vi "Read & Graph Measurement File.vi"() -> ()   [LabVIEW 2019]
panel:
  in  "File 2":path=path "test.tdms" caption="Filename"
  out "Signals 2":dynamicdata(graph) caption="Signals"
  in  "File 1":path=path "test.tdms" caption="Filename"
  out "Signals 1":dynamicdata(graph) caption="Signals"
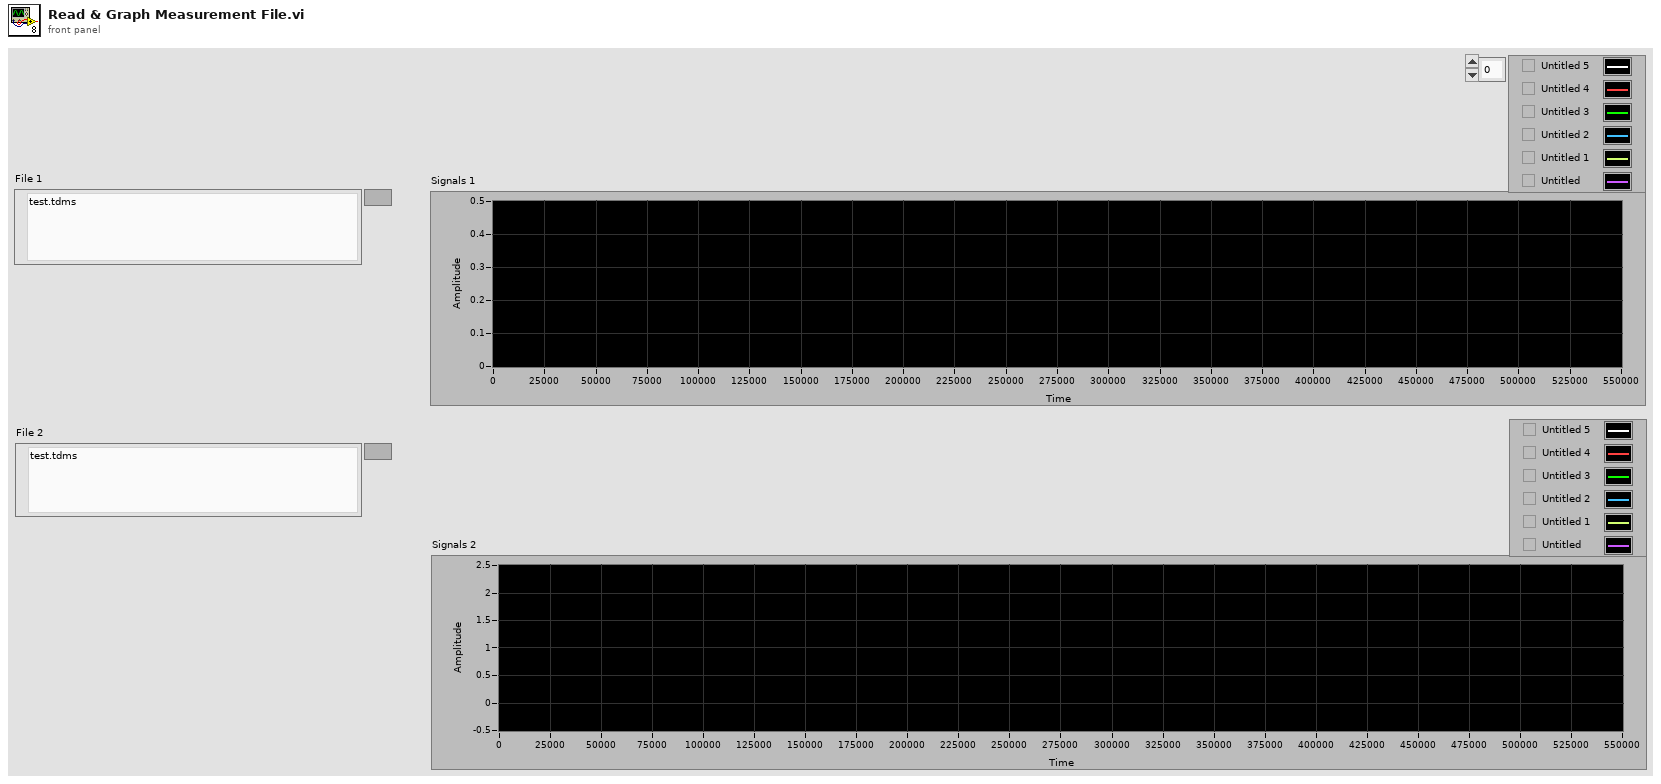
[diagram p1: front panel]
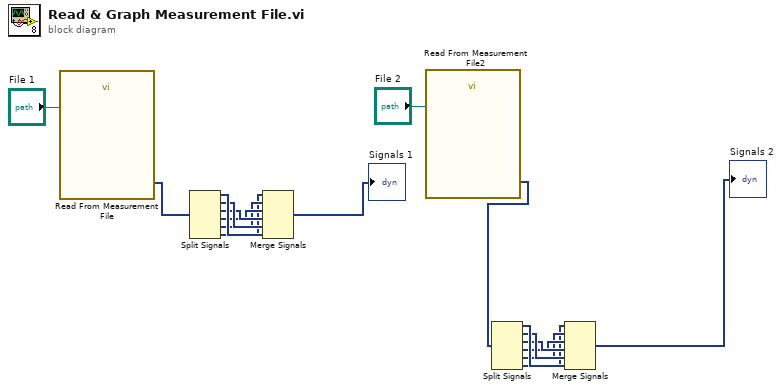
[diagram p0: block diagram]
diagram:
  n1 = call "Read From Measurement File"("Filename"="File 1") -> ("Signals"=w16:dynamicdata)  [unwired: 5 in, 5 out]
  n2 = Split Signals(w16) -> (w15:dynamicdata, w14:dynamicdata, w13:dynamicdata, w12:dynamicdata, w11:dynamicdata, w10:dynamicdata)  [unwired: 6 in]
  n3 = Merge Signals(w10, w11, w12, w13, w14, w15) -> (→"Signals 1":dynamicdata)
  n4 = call "Read From Measurement File2"("Filename"="File 2") -> ("Signals"=w2:dynamicdata)  [unwired: 5 in, 5 out]
  n5 = Split Signals(w2) -> (w8:dynamicdata, w7:dynamicdata, w6:dynamicdata, w5:dynamicdata, w4:dynamicdata, w3:dynamicdata)  [unwired: 6 in]
  n6 = Merge Signals(w3, w4, w5, w6, w7, w8) -> (→"Signals 2":dynamicdata)
